vi "Sequence.Test.RoteateProducts.vi"(8 "error in (no error)":errorcluster, 9 "TS":timestamp, 10 "Status.Prod in":T1[](array[typedef])) -> (0 "error out":errorcluster, 2 "Status.Prod out":T1[](array[typedef]), 3 "Status Prev":T1)   [LabVIEW 2016]
uses:
  Sequence.Test.BreakReason.ctl
  Sequence.Step.Status.ctl
  Sequence.Prod.StatusData.ctl
  Station/Station.ProductSlot.ctl
  Sequence.SerialsFglb.SerialData.ctl
  Sequence.SerialsFglb.Action.ctl
  Global/ApplicationGlobal.vi
  Sequence.Test.Unload.Status.ctl
  Sequence.Slot.StatusData.ctl
  Sequence.Test.Status.ctl
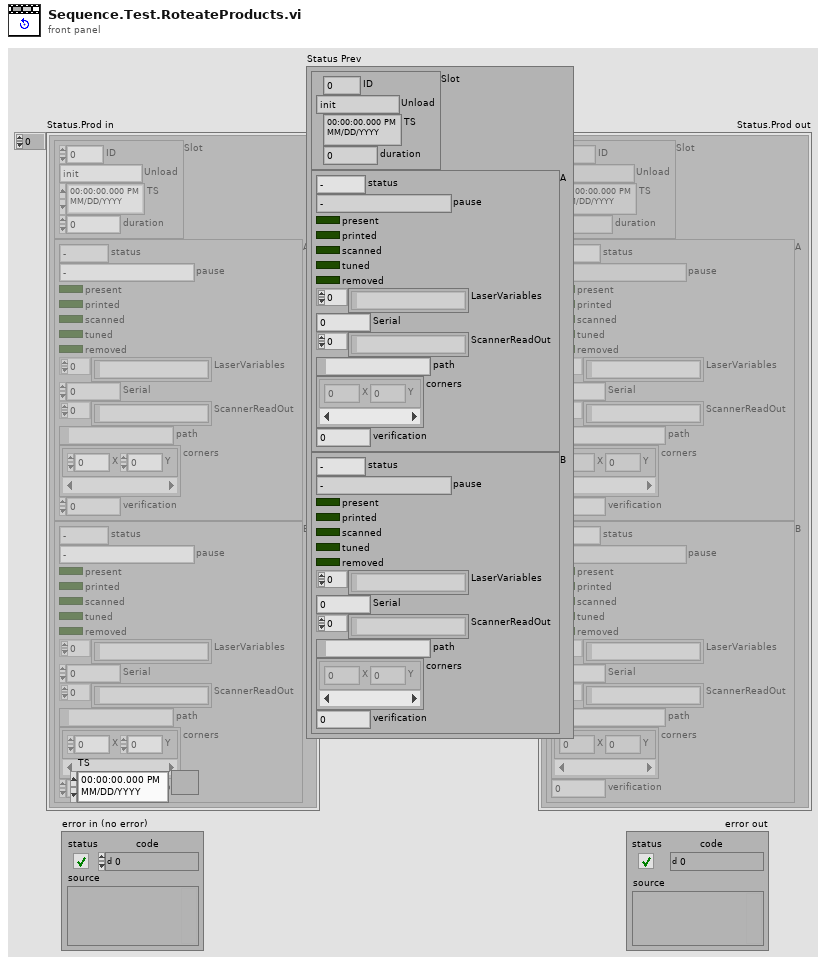
[diagram p1: front panel]
types:
  T1 = typedef "Sequence.Test.Status.ctl" = cluster{"Slot":T2, "A":T4, "B":T4}
  T2 = typedef "Sequence.Slot.StatusData.ctl" = cluster{"ID":i32, "Unload":T3, "TS":timestamp, "duration":u32}
  T3 = typedef "Sequence.Test.Unload.Status.ctl" = enum16{"init", "check NOK", "check OK", "wait on NOK", "wait on OK", "wait on Unload", "done"}
  T4 = typedef "Sequence.Prod.StatusData.ctl" = cluster{"status":T5, "pause":T6, "present":bool, "printed":bool, "scanned":bool, "tuned":bool, "removed":bool, "LaserVariables":string[], "Serial":i32, "ScannerReadOut":string[], "path":path, "corners":cluster{"X":i32, "Y":i32}[], "verification":u8}
  T5 = typedef "Sequence.Step.Status.ctl" = enum16{"-", "Pending", "Running", "Skipped", "Passed", "Failed", "Done", "Error", "Aborted", "Stopped"}
  T6 = typedef "Sequence.Test.BreakReason.ctl" = enum16{"-", "NOK container", "OK container", "Rev empty", "Rev missing", "Rev wrong", "Fork missing", "Fork wrong", "NOK limit", "Unload failure", "Single slot", "Part done", "Err: Prod move work", "Err: Prod move home", "Err: Prod lift work", "Err: Prod lift home", "Err: Prod Arm Work", "Err: Prod Arm NOK", "Err: Prod Arm OK", "Err: Prod NOK suck", "Err: Prod NOK drop", "Err: Prod OK missing", "Err: Prod OK suck", "Err: Prod OK drop"}
  T7 = typedef "Sequence.SerialsFglb.SerialData.ctl" = cluster{"TS":timestamp, "Slot":T8, "Serial":i32, "Global":bool}
  T8 = typedef "Station.ProductSlot.ctl" = enum8{"A", "B"}
  T9 = typedef "Sequence.SerialsFglb.Action.ctl" = enum16{"init", "get", "get next", "pass", "fail", "confirm", "clean"}
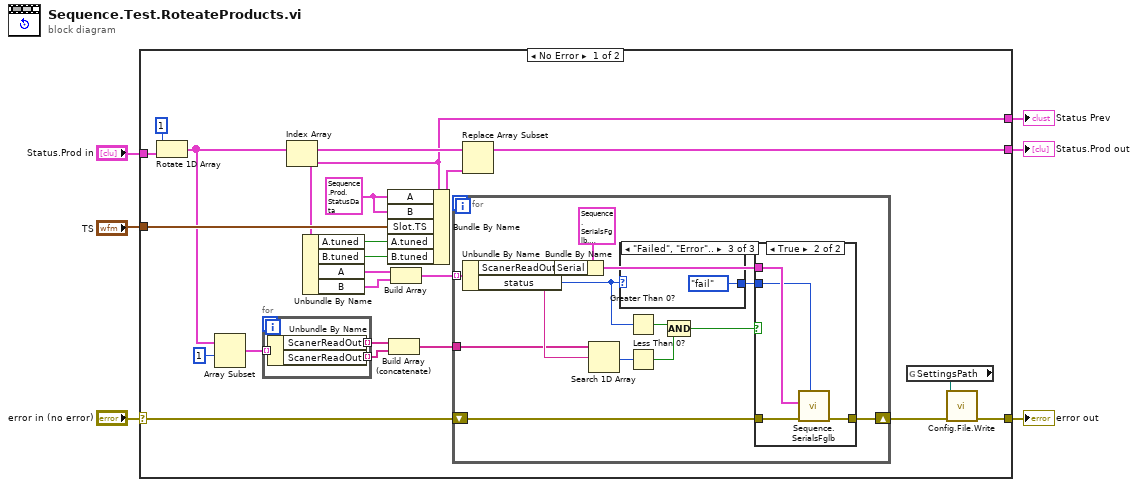
[diagram p0: block diagram]
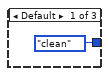
[diagram p2: hidden frame]
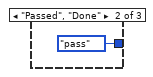
[diagram p3: hidden frame]
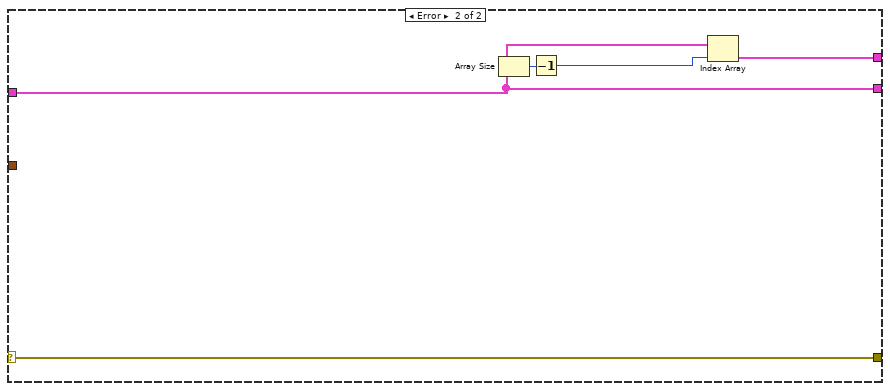
[diagram p5: hidden frame]
diagram:
  n1 = case shown="No Error" "error in (no error)" {
    selector: "error in (no error)" -> [w15 w57]
    tunnel: "Status.Prod in" -> [w25 w55]
    tunnel: [w12 w57] -> w5
    tunnel: "TS" -> [w21 _]
    tunnel: [w7 w56] -> w3
    tunnel: [w24 w55] -> w1
    frame No Error {
      w28 = T4 {"status"=enum."-", "pause"=enum."-", "present"=FALSE, "printed"=FALSE, "scanned"=FALSE, "tuned"=FALSE, "removed"=FALSE, "LaserVariables"=[], "Serial"=0, "ScannerReadOut"=[], "path"=path "", "corners"=[], "verification"=0} ("A")
      n2 = Rotate 1D Array(1:w25, 2:1 ("n")) -> (0:w20:T1[])
      n3 = Array Subset(array=w20, index=1) -> (w18:T1[])  [unwired: 1 in]
      n4 = for {
        tunnel: w18 -> [w31] mode=indexing
        tunnel: [w30] -> w17 mode=indexing
        tunnel: [w29] -> w16 mode=indexing
        n5 = Unbundle By Name(w31) -> ("ScanerReadOut"=w30:string, "ScanerReadOut"=w29:string)
      }
      n6 = Index Array(array=w20) -> (element=w7:T1)  [unwired: 1 in]
      n7 = Unbundle By Name(w7) -> ("A.tuned"=w26:bool, "B.tuned"=w27:bool, "A"=w10:T4, "B"=w8:T4)
      n8 = Bundle By Name(cluster=w7, "A"=w28, "B"=w28, "Slot.TS"=w21, "A.tuned"=w26, "B.tuned"=w27) -> (w23:T1)
      n9 = Build Array (concatenate)(w17, w16) -> (w11:string[])
      n10 = Build Array(w10, w8) -> (w9:T4[])
      n11 = for {
        shift-right: [w43] -> w13
        shift-left: w15 -> [w44]
        tunnel: w9 -> [w41] mode=indexing
        tunnel: w11 -> [w35]
        n12 = Unbundle By Name(w41) -> ("ScanerReadOut"=w36:string, "status"=w38:T5)
        n13 = Bundle By Name(cluster=T7 {"TS"=timestamp(0 s since 1904-01-01), "Slot"=enum."A", "Serial"=0, "Global"=FALSE} ("Serial data in"), "Serial"=w36) -> (w40:T7)
        n14 = Search 1D Array(1D array=w35, element=w36) -> (index of element=w37:i32)  [unwired: 1 in]
        n15 = case shown="\"Failed\", \"Error\".." w38 {
          tunnel: [Sequence.SerialsFglb.Action."clean" ("Action (get)") Sequence.SerialsFglb.Action."pass" ("Action (get)") Sequence.SerialsFglb.Action."fail" ("Action (get)")] -> w39
          frame Default {
          }
          frame "Passed", "Done" {
          }
          frame "Failed", "Error".. {
          }
        }
        n16 = Greater Than 0?(x=w38) -> (x > 0?=w34:bool)
        n17 = Less Than 0?(x=w37) -> (x < 0?=w33:bool)
        n18 = Compound Arithmetic op=AND(w34, w33) -> (w32:bool)
        n19 = case shown="True" w32 {
          tunnel: w44 -> [w48 w52]
          tunnel: [w48 w51] -> w43
          tunnel: w40 -> [_ w50]
          tunnel: w39 -> [_ w49]
          frame False {
          }
          frame True {
            n20 = call "Sequence.SerialsFglb.vi"("Action (get)"=w49, "error in"=w52, "Serial data in"=w50) -> ("error out"=w51:errorcluster)  [unwired: 4 in, 4 out]
          }
        }
      }
      n21 = Replace Array Subset(array=w20, new element=w23) -> (w24:T1[])  [unwired: 1 in]
      n22 = global read "ApplicationGlobal.vi" "SettingsPath"() -> (w14:path)
      n23 = call "Config.File.Write.vi"("error in"=w13, "path"=w14) -> ("error out"=w12:errorcluster)  [unwired: 9 in]
    }
    frame Error {
      n24 = Array Size(array=w55) -> (size(s)=w54:i32)
      n25 = Decrement(x=w54) -> (x-1=w53:i32)
      n26 = Index Array(array=w55, index=w53) -> (element=w56:T1)
    }
  }
  "Status.Prod out" <- w1
  "error out" <- w5
  "Status Prev" <- w3
